vi "Launch Test.vi"(8 "error in (no error)":errorcluster, 10 "Test Name":string, 11 "Test Application Controller in":refnum<class "Test Application Controller.lvclass">) -> (0 "error out":errorcluster, 3 "Test Application Controller out":refnum<class "Test Application Controller.lvclass">)   [LabVIEW 2017, in "Test Application Controller.lvlib" / "Test Application Controller.lvclass"]
uses:
  Test Application Controller.lvclass
  C:/Program Files (x86)/National Instruments/LabVIEW 2017/vi.lib/ActorFramework/Actor/Actor.lvclass
  Test Application Controller Messages/New Test Window Launched Msg/New Test Window Launched Msg.lvclass
  D:/Career/Tesla/LabVIEW_Interview_Problem/Tesla Test Application/Test/Test Messages/Test Window Launched Msg/Test Window Launched Msg.lvclass
  Test Application Controller Messages/Status String Msg/Status String Msg.lvclass
  D:/Career/Tesla/LabVIEW_Interview_Problem/Tesla Test Application/Test/Test Messages/Send Status String Msg/Status String Msg.lvclass
  Test Application Controller Messages/Test Progress Msg/Test Progress Msg.lvclass
  D:/Career/Tesla/LabVIEW_Interview_Problem/Tesla Test Application/Test/Test Messages/Test Progress Msg/Test Progress Msg.lvclass
  Test Application Controller.lvclass/Test Application Controller.ctl
  Test/Test/Test.lvclass
  Text based Communications Test/Text based Communications Test.lvclass
  D:/Career/Tesla/LabVIEW_Interview_Problem/Tesla Test Application/Test/Test/Test.lvclass
  Protocol Verification Test/Protocol Verification Test.lvclass
  Network Test/Network Test.lvclass
  Test/Test/Test.lvclass/Test.ctl
  <vilib>/ActorFramework/Actor/Actor.lvclass
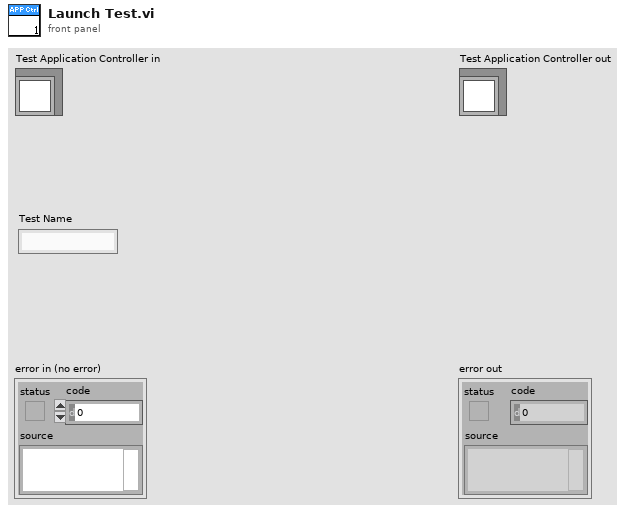
[diagram p1: front panel]
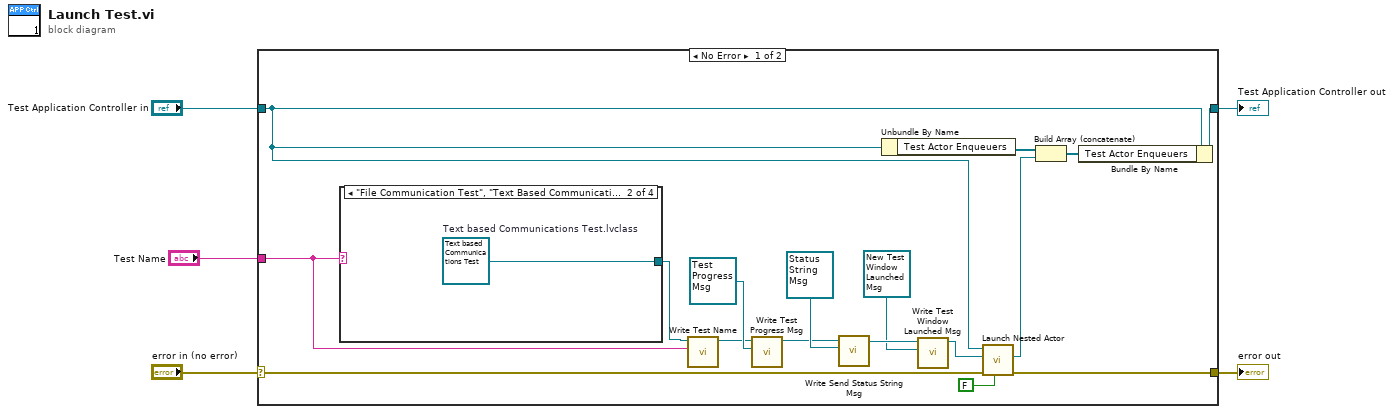
[diagram p0: block diagram]
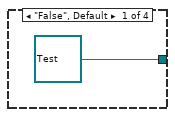
[diagram p2: hidden frame]
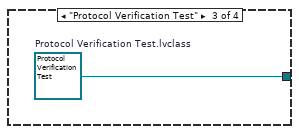
[diagram p3: hidden frame]
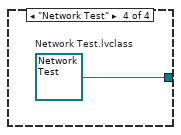
[diagram p4: hidden frame]
diagram:
  n1 = case shown="No Error" "error in (no error)" {
    selector: "error in (no error)" -> [w19 w28]
    tunnel: [w18 w28] -> w4
    tunnel: [w17 w27] -> w2
    tunnel: "Test Application Controller in" -> [w16 w27]
    tunnel: "Test Name" -> [w6 _]
    frame No Error {
      n2 = case shown="\"File Communication Test\", \"Text Based Communication Test\"" w6 {
        tunnel: [refnum<class "Test.lvclass"> refnum ("Test in") w24 w25 w26] -> w8
        frame "False", Default {
        }
        frame "File Communication Test", "Text Based Communication Test" {
          w24 = refnum<class "Text based Communications Test.lvclass"> refnum  # Text based Communications Test.lvclass
        }
        frame "Protocol Verification Test" {
          w25 = refnum<class "Protocol Verification Test.lvclass"> refnum  # Protocol Verification Test.lvclass
        }
        frame "Network Test" {
          w26 = refnum<class "Network Test.lvclass"> refnum  # Network Test.lvclass
        }
      }
      n3 = call-dynamic "Write Test Name.vi"("Test Name"=w6, "Test in"=w8) -> ("Test out"=w7:refnum<class "Test.lvclass">)  [unwired: 8 in, 1 out]
      n4 = call "Write Test Progress Msg.vi"("Test.lvlib:Test Progress Msg.lvclass"=refnum<class "Test Progress Msg.lvclass"> refnum ("Test Application Controller.lvlib:Test Progress Msg.lvclass"), "Test in"=w7) -> ("Test out"=w10:refnum<class "Test.lvclass">)  [unwired: 9 in]
      n5 = call "Write Send Status String Msg.vi"("Test.lvlib:Send Status String Msg.lvclass"=refnum<class "Status String Msg.lvclass"> refnum ("Test Application Controller.lvlib:Status String Msg.lvclass"), "Test in"=w10) -> ("Test out"=w22:refnum<class "Test.lvclass">)  [unwired: 9 in]
      n6 = Unbundle By Name(w16) -> ("Test Actor Enqueuers"=w15:refnum<class "Message Enqueuer.lvclass">[])
      n7 = call "Write Test Window Launched Msg.vi"("Test.lvlib:Test Window Launched Msg.lvclass"=refnum<class "New Test Window Launched Msg.lvclass"> refnum ("Test Application Controller.lvlib:New Test Window Launched Msg.lvclass"), "Test in"=w22) -> ("Test out"=w21:refnum<class "Test.lvclass">)  [unwired: 9 in]
      n8 = call <vilib>:"Launch Nested Actor.vi"("Open Actor Core front panel? (F)"=FALSE, "error in (no error)"=w19, "Nested Actor"=w21, "Caller Actor in"=w16) -> ("error out"=w18:errorcluster, "Nested Actor's Enqueuer"=w14:refnum<class "Message Enqueuer.lvclass">)  [unwired: 5 in, 1 out]
      n9 = Build Array (concatenate)(w15, w14) -> (w13:refnum<class "Message Enqueuer.lvclass">[])
      n10 = Bundle By Name(cluster=w16, "Test Actor Enqueuers"=w13) -> (w17:refnum<class "Test Application Controller.lvclass">)
    }
    frame Error {
    }
  }
  "error out" <- w4
  "Test Application Controller out" <- w2
